vi "Create.vi"(8 "error in (no error)":errorcluster, 9 "Image Size":T1, 11 "Camera Parameters":T2) -> (0 "error out":errorcluster, 3 "Image Distorter":refnum<class "Image Distorter.lvclass">)   [LabVIEW 2020, in "image.lvlib" / "Image Distorter.lvclass"]
doc: "Create a New Image Distorter with the given Camera Parameters"
uses:
  Image Distorter.lvclass
  common/Camera Parameters.ctl
  common/Camera Matrix.ctl
  common/Camera Distortion Coefficients.ctl
  common/Image Size (Integer).ctl
  Image Distorter.lvclass/Image Distorter.ctl
  common/common.lvlib
  common/bin/gartoolkit_32-1.dll
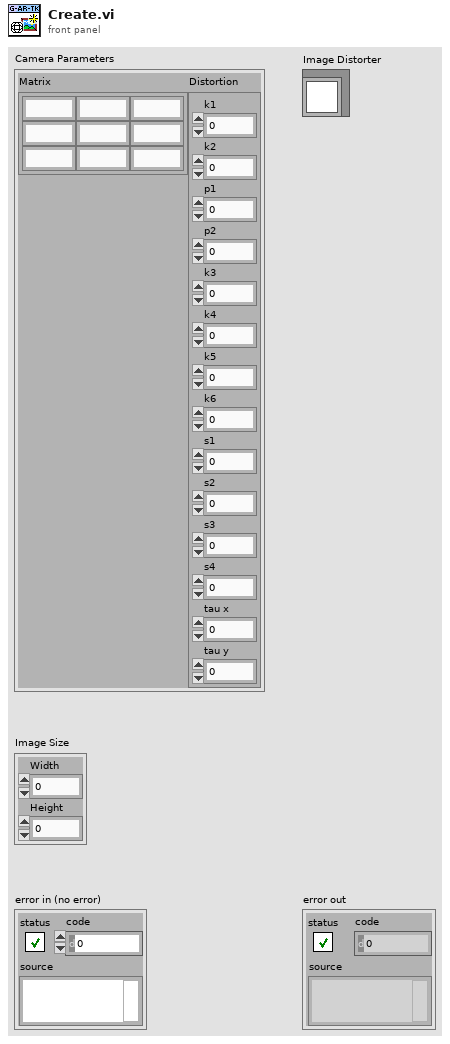
[diagram p1: front panel]
types:
  T1 = typedef "common.lvlib/Image Size (Integer).ctl" = cluster{"Width":u16, "Height":u16}
  T2 = typedef "common.lvlib/Camera Parameters.ctl" = cluster{"Matrix":T3, "Distortion":T4}
  T3 = typedef "common.lvlib/Camera Matrix.ctl" = cluster{"m 0,0":dbl, "m 0,1":dbl, "m 0,2":dbl, "m 1,0":dbl, "m 1,1":dbl, "m 1,2":dbl, "m 2,0":dbl, "m 2,1":dbl, "m 2,2":dbl}
  T4 = typedef "common.lvlib/Camera Distortion Coefficients.ctl" = cluster{"k1":dbl, "k2":dbl, "p1":dbl, "p2":dbl, "k3":dbl, "k4":dbl, "k5":dbl, "k6":dbl, "s1":dbl, "s2":dbl, "s3":dbl, "s4":dbl, "tau x":dbl, "tau y":dbl}
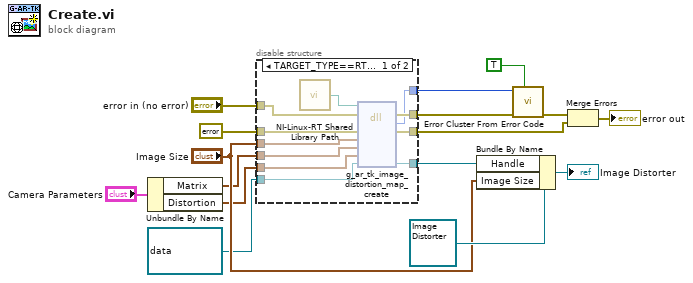
[diagram p0: block diagram]
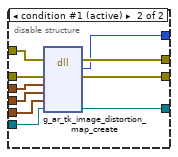
[diagram p2: hidden frame]
diagram:
  n1 = Unbundle By Name("Camera Parameters") -> ("Matrix"=w8:T3, "Distortion"=w7:T4)
  n2 = disable-structure shown="TARGET_TYPE==RT&&OS==Linux" {
    disable-tunnel: "error in (no error)" -> [w27 w37]
    disable-tunnel: errorcluster {"status"=FALSE, "code"=0, "source"=""} ("error constant") -> [w26 w36]
    disable-tunnel: "Image Size" -> [w25 w35]
    disable-tunnel: w8 -> [w24 w34]
    disable-tunnel: w7 -> [w23 w33]
    disable-tunnel: refnum<data-value> refnum ("EDVR") -> [w22 w32]
    disable-tunnel: [w21 w31] -> w5
    disable-tunnel: [w20 w30] -> w4
    disable-tunnel: [w19 w29] -> w3
    disable-tunnel: [w18 w28] -> w2
    frame condition #0 {
      n3 = call "NI-Linux-RT Shared Library Path.vi"() -> ("Path"=w17:path)
      n4 = dll-call lib="C:/serenial/libraries/g-augmented-reality-toolkit/LabVIEW/g_ar_toolkit.common/bin/g_ar_toolkit.1.32.dll" fn="g_ar_tk_image_distortion_map_create" ("g_ar_toolkit.*.*:g_ar_tk_image_add_weighted")(path in=w17, error in=w27, "error_cluster"=w26, "size"=w25, "camera_matrix"=w24, "distortion_param"=w23, "EDVR"=w22) -> (error out=w21:errorcluster, w20:i32, "error_cluster"=w19:errorcluster, "EDVR"=w18:refnum<data-value>)  [unwired: 4 in, 1 out]
    }
    frame condition #1 (active) {
      n5 = dll-call lib="C:/serenial/lib/g-augmented-reality-toolkit/LabVIEW/common/bin/gartoolkit_*-1.*" fn="g_ar_tk_image_distortion_map_create" ("g_ar_toolkit.*.*:g_ar_tk_image_add_weighted")(error in=w37, "error_cluster"=w36, "size"=w35, "camera_matrix"=w34, "distortion_param"=w33, "EDVR"=w32) -> (error out=w31:errorcluster, w30:i32, "error_cluster"=w29:errorcluster, "EDVR"=w28:refnum<data-value>)  [unwired: 5 in, 1 out]
    }
  }
  n6 = Bundle By Name(cluster=refnum<class "Image Distorter.lvclass"> refnum ("Image Rectifier out"), "Handle"=w2, "Image Size"="Image Size") -> (→"Image Distorter":refnum<class "Image Distorter.lvclass">)
  n7 = call <vilib>:"Error Cluster From Error Code.vi"("show call chain? (False)"=TRUE, "error in (no error)"=w5, "error code (0)"=w4) -> ("error out"=w16:errorcluster)  [unwired: 6 in]
  n8 = Merge Errors(w16, w3) -> (→"error out":errorcluster)
